vi "LDA_Beam_Alignment.vi"() -> ()   [LabVIEW 2017]
uses:
  Anemometry Sub Vis/Controls/Beam_Type.ctl
  Anemometry Sub Vis/Gen Trav/Traverse_cluster.ctl
  Anemometry Sub Vis/Gen Trav/Spacing.ctl
  Anemometry Sub Vis/Controls/Multi_run_mode.ctl
  Anemometry Sub Vis/Controls/User_Specific_mode.ctl
  Anemometry Sub Vis/Controls/Tunnel_Coordinates.ctl
  Anemometry Sub Vis/Controls/Post_Process.ctl
  Anemometry Sub Vis/Controls/Setup.ctl
  Anemometry Sub Vis/Gen Trav/Trav_mode.ctl
  Anemometry Sub Vis/Globals/Trav_pos_global.vi
  Anemometry Sub Vis/Globals/Meas_global.vi
  Anemometry Sub Vis/Globals/Preference_global.vi
panel:
  in  "Beams to peak":bool[](array[boolean])=[TRUE, TRUE, TRUE, TRUE]
  out "Beam Names":string[](array[string])
  out "Probe is facing...":string
  out "In-Plane Roll (deg)":dbl
  out "Pitch (deg)":dbl
  out "Yaw (deg)":dbl
  out "Vp (Actual Probe dir. vect)":dbl[](array[numeric])
  in  "Mode":T1(ring)
  out "Values Out":dbl[][](array[numeric])
  out "Original Position":dbl[](array[numeric]) format="%.2f"
  in  "Traverse Position":dbl[](array[numeric])=[0.0, 0.0, 0.0] format="%.2f"
  out "Message":string
  in  "Go Back":bool
  in  "OK":bool
  in  "stop":bool
  in  "Working On":T2 items=["Green Unshifted", "Green Shifted", "Blue Unshifted", "Blue Shifted"]
  # "X                 Y              Z"
  # "X                 Y              Z"
  # "Green Unshifted\nGreen Shifted\nBlue Unshifted\nBlue Shifted"
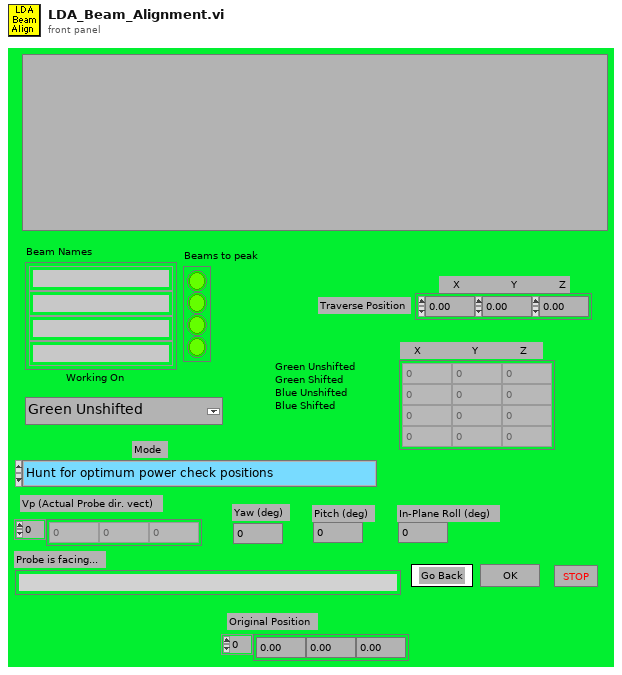
[diagram p1: front panel]
types:
  T1 = enum16{"Hunt for optimum power check positions", "Check Beam powers now", "Peak up beam power using manipulators"}
  T2 = typedef "Beam_Type.ctl" = u16
  T3 = typedef "Traverse_cluster.ctl" = cluster{"Start X":sgl, "Start Y":sgl, "Start Z":sgl, "End X":sgl, "End Y":sgl, "End Z":sgl, "No. of pts.":i32, "Spacing":T4, "Filename":path, "Tunnel Speed":dbl, "Averaging time (min)":dbl, "Extra Commands":string, "Carrier_1 Q (l/min)":dbl, "Carrier_2 Q (l/min)":dbl, "Trace Gas Concentration (%)":dbl, "Specific Arguments":string, "Comments":string, "Row No":i32, "Row Type Selector":T5, "Completion time":string, "Row Duration (mins)":dbl, "No. of Valid pts.":i32, "Meas Setup File":string}
  T4 = typedef "Spacing.ctl" = enum16{"Linear", "Log", "Gauss", "Specified", "N/A"}
  T5 = typedef "Multi_run_mode.ctl" = enum16{"Move Traverse Only", "Set Tunnel Speed Only", "Set Source Only", "Set Measurement Conditions", "Single Measurement", "Vertical Profile", "Lateral Profile", "Longitudinal Profile", "Explore Volume", "Multi-Axis Profile", "Auto Calibrate", "Meas Fast FID Bkgnd", "Check Beam Power", "Scanning Valve Measurement", "Run VI Named:", "Set ADAM Ch", "Wait (minutes)", "Send Message", "Synchronize With:", "Fall Back to this Row", "Turn Off Row Repeating", "Blank Row", "Traverse 3D Volume"}
  T6 = typedef "Tunnel_Coordinates.ctl" = enum16{"Work in Tunnel Coordinates", "Work in Model Coordinates"}
  T7 = typedef "User_Specific_mode.ctl" = enum16{"Check VI only", "Run VI"}
  T8 = typedef "Post_Process.ctl" = enum16{"Take New Data", "Post Process Raw Data File"}
  T9 = enum16{"Load setup from excel file", "Save setup to excel file"}
  T10 = enum16{"Load From Excel File", "Save to Excel File"}
  T11 = typedef "Setup.ctl" = enum16{"Run Program", "Show Setup", "Save Current Setup", "Setup Front Panel"}
  T12 = typedef "Trav_mode.ctl" = enum16{"Move traverse", "Read traverse position", "Teach Position"}
  T13 = typedef "LDA_Beam_Cluster.ctl" = cluster{"Vg1 (Green 1 dir. vect.)":dbl[], "Vg2  (Green 2 dir. vect.)":dbl[], "Vb1 (Blue 1 dir. vect.)":dbl[], "Vb2 (Blue 1 dir. vect.)":dbl[], "Porb (Orb XYZ posn. forced coplanar)":dbl[], "Porb (Orb XYZ posn. - allow skew)":dbl[], "Orb posn. uncertainty, +/- dx, dy, dz":dbl[], "Vp (Actual Probe dir. vect)":dbl[], "Yaw (deg)":dbl, "Pitch (deg)":dbl, "In-Plane Roll (deg)":dbl, "Beam Half Angle (deg)":dbl, "B1 Close P11":dbl[], "B1 Far P12":dbl[], "B2 Close P22":dbl[], "B2 Far P21":dbl[], "Projected Roll (deg)":dbl, "Green Velocity Vector":dbl[], "Blue Velocity Vector":dbl[], "Probe is facing....":string, "Calculation Method":string}
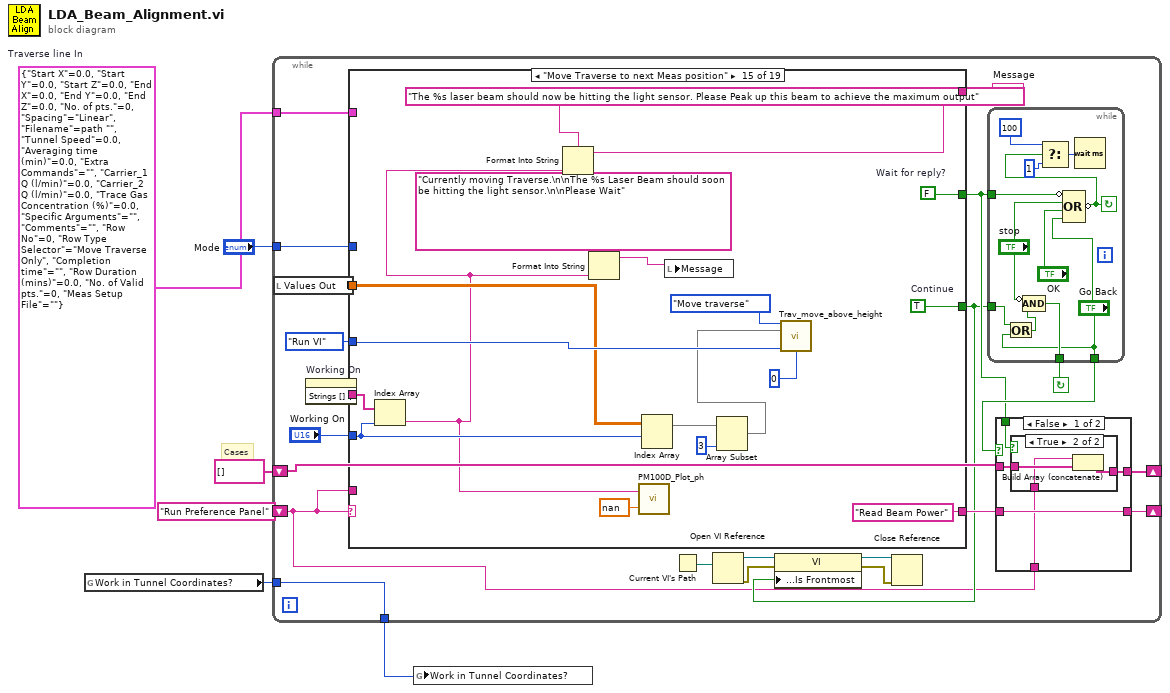
[diagram p0: block diagram]
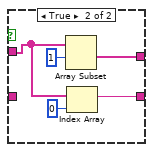
[diagram p3: hidden frame]
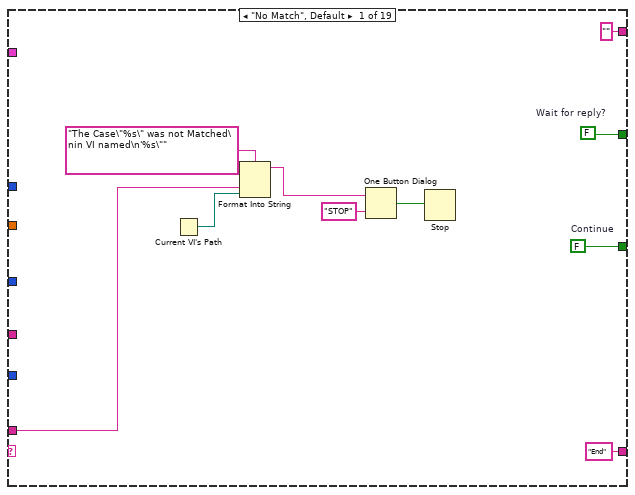
[diagram p4: hidden frame]
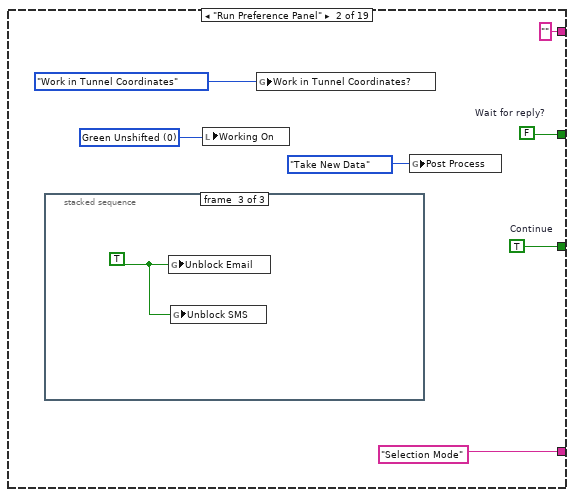
[diagram p5: hidden frame]
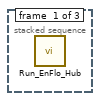
[diagram p6: hidden frame]
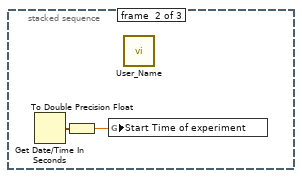
[diagram p7: hidden frame]
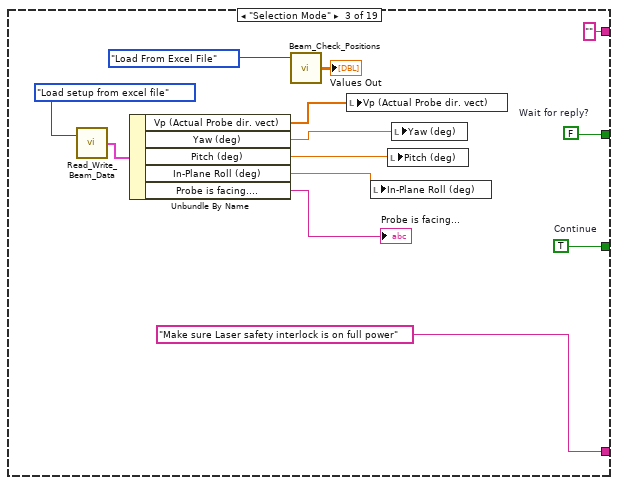
[diagram p8: hidden frame]
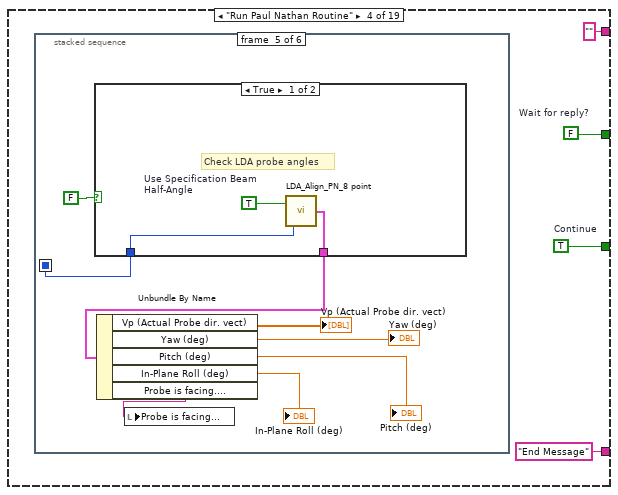
[diagram p9: hidden frame]
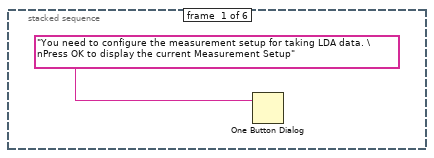
[diagram p10: hidden frame]
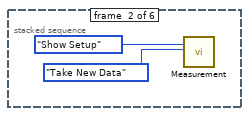
[diagram p11: hidden frame]
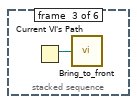
[diagram p12: hidden frame]
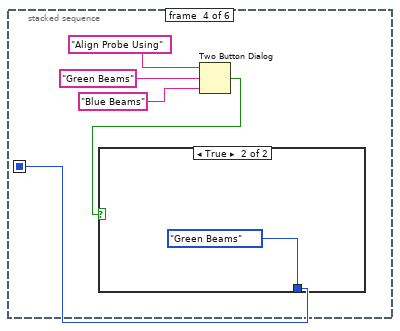
[diagram p13: hidden frame]
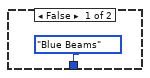
[diagram p14: hidden frame]
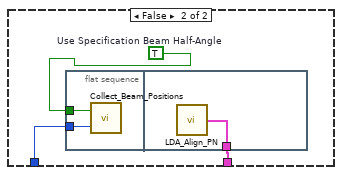
[diagram p15: hidden frame]
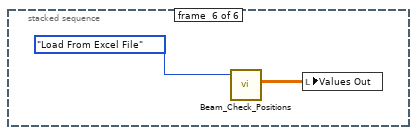
[diagram p16: hidden frame]
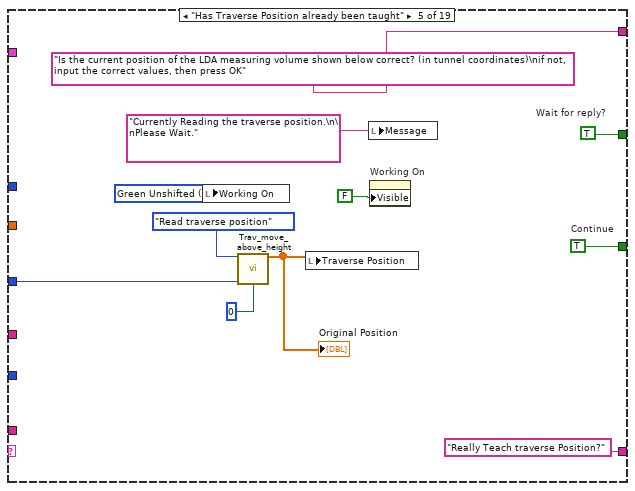
[diagram p17: hidden frame]
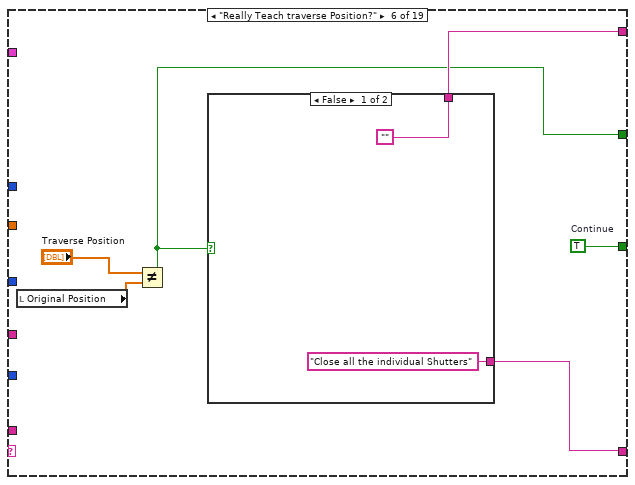
[diagram p18: hidden frame]
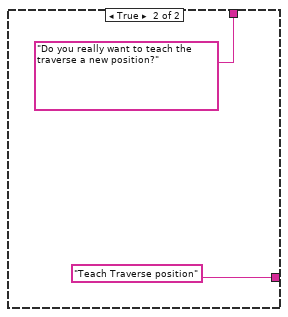
[diagram p19: hidden frame]
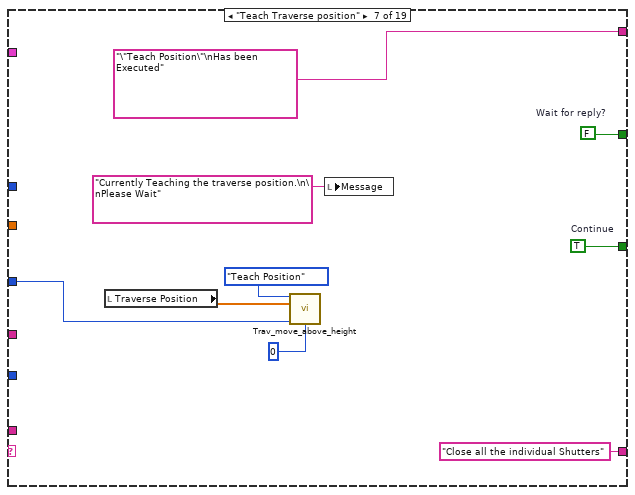
[diagram p20: hidden frame]
diagram:
  w3 = T3 {"Start X"=0.0, "Start Y"=0.0, "Start Z"=0.0, "End X"=0.0, "End Y"=0.0, "End Z"=0.0, "No. of pts."=0, "Spacing"=enum."Linear", "Filename"=path "", "Tunnel Speed"=0.0, "Averaging time (min)"=0.0, "Extra Commands"="", "Carrier_1 Q (l/min)"=0.0, "Carrier_2 Q (l/min)"=0.0, "Trace Gas Concentration (%)"=0.0, "Specific Arguments"="", "Comments"="", "Row No"=0, "Row Type Selector"=enum."Move Traverse Only", "Completion time"="", "Row Duration (mins)"=0.0, "No. of Valid pts."=0, "Meas Setup File"=""}  # Traverse line In
  # "Cases"
  n1 = global read "Trav_pos_global.vi" "Work in Tunnel Coordinates?"() -> (w1:T6)
  n2 = while {
    tunnel: w3 -> [w9]
    tunnel: "Mode" -> [w10]
    shift-left: string[] [] -> [w26]
    shift-right: [w25] -> _
    shift-left: "Run Preference Panel" -> [w8]
    shift-right: [w24] -> _
    tunnel: [w7] -> w2
    tunnel: w1 -> [w7]
    stop <- w28 continue-if-true
    n3 = local read "Values Out"() -> (w11:dbl[][])
    n4 = property on="Working On" class="Ring (strict)"() -> ("Strings []"=w13:string[])  [unwired: 2 in, 2 out]
    n5 = case shown="\"Move Traverse to next Meas position\"" w8 {
      tunnel: [w63 w70 w86 w90 w131 w137 w150 w160 w169 w185 w210 w219 w233 w259 w280 w284 w299 w307 w317] -> w14
      tunnel: ["End" "Selection Mode" "Make sure Laser safety interlock is on full power" "End Message" "Really Teach traverse Position?" w132 "Close all the individual Shutters" "Manually move the traverse using hand wheels" "Read traverse position" w173 w204 "Hunt for optimum power check positions" "End Message" "End Message" "Read Beam Power" "Save measured beam Power" w291 "End Message" "End"] -> w23
      tunnel: [w62 w69 w85 w89 w130 w133 w149 w159 w168 w184 w209 w218 w234 w260 w279 w283 w298 w306 w316] -> w15
      tunnel: ["" "" "" "" "Is the current position of the LDA measuring volume shown below correct? (in tunnel coordinates)\nif not, input the correct values, then press OK" w136 "\"Teach Position\"\nHas been Executed" w153 w162 w170 "Make sure the Laser safety interlock is on full power and all the shutters are open." "Please select which beams you would like to hunt for optimum power check positions for by pressing the green buttons." "" "" w266 w282 w290 "Now open all the individual shutters so all four beam are showing." w310] -> w22
      tunnel: User_Specific_mode."Run VI" ("Simulate/Run") -> [_ _ _ _ w126 _ w145 _ _ w181 _ _ _ _ w276 _ _ _ _]
      tunnel: w13 -> [_ _ _ _ _ _ _ w158 w165 _ w207 w214 w222 _ w271 _ w287 _ _]
      tunnel: "Working On" -> [_ _ _ _ _ _ _ w157 w164 w172 w206 _ _ _ w270 _ w288 _ _]
      tunnel: w11 -> [_ _ _ _ _ _ _ _ _ w171 _ _ _ _ w269 _ w296 _ _]
      tunnel: w10 -> [_ _ _ _ _ _ _ _ _ _ w205 _ _ _ _ _ _ _ w313]
      tunnel: w9 -> [_ _ _ _ _ _ _ _ _ _ _ _ _ w257 _ _ _ _ _]
      tunnel: w8 -> [w54 _ _ _ _ _ _ _ _ _ _ _ _ _ _ _ _ _ _]
      frame "No Match", Default {
        w62 = FALSE  # Wait for reply?
        w63 = FALSE  # Continue
        n6 = Current VI's Path() -> (path=w55:path)
        n7 = Format Into String(format string="The Case\"%s\" was not Matched\nin VI named\n'%s\"" ("Format String"), w54, w55) -> (resulting string=w58:string)  [unwired: 2 in, 1 out]
        n8 = One Button Dialog(message=w58, button name ("OK")="STOP") -> (true=w56:bool)
        n9 = Stop(stop? (T)=w56) -> ()
      }
      frame "Run Preference Panel" {
        w67 = T2 0 items=["Green Unshifted", "Green Shifted", "Blue Unshifted", "Blue Shifted"] ("Beam Type")
        w69 = FALSE  # Wait for reply?
        w70 = TRUE  # Continue
        n10 = stacked-sequence {
          frame #0 {
            n11 = call "Run_EnFlo_Hub.vi"() -> ()  [unwired: 1 in, 7 out]
          }
          frame #1 {
            n12 = Get Date/Time In Seconds() -> (seconds since 1Jan1904=w72:timestamp)
            n13 = To Double Precision Float(number=w72) -> (double precision float=w71:dbl)
            n14 = global write "Meas_global.vi" "Start Time of experiment"(w71) -> ()
            n15 = call "User_Name.vi"() -> ()  [unwired: 1 out]
          }
          frame #2 {
            w73 = TRUE
            n16 = global write "Preference_global.vi" "Unblock Email"(w73) -> ()
            n17 = global write "Preference_global.vi" "Unblock SMS"(w73) -> ()
          }
        }
        n18 = local write "Working On"(w67) -> ()
        n19 = global write "Trav_pos_global.vi" "Work in Tunnel Coordinates?"(Tunnel_Coordinates."Work in Tunnel Coordinates" ("Work in Tunnel Coordinates?")) -> ()
        n20 = global write "Meas_global.vi" "Post Process"(Post_Process."Take New Data" ("Post Process")) -> ()
      }
      frame "Selection Mode" {
        w85 = FALSE  # Wait for reply?
        w86 = TRUE  # Continue
        n21 = call "Read_Write_Beam_Data.vi"("Mode"=T9."Load setup from excel file") -> ("Beam Data Out"=w75:T13)  [unwired: 1 in]
        n22 = Unbundle By Name(w75) -> ("Vp (Actual Probe dir. vect)"=w80:dbl[], "Yaw (deg)"=w77:dbl, "Pitch (deg)"=w78:dbl, "In-Plane Roll (deg)"=w79:dbl, "Probe is facing...."=→"Probe is facing...":string)
        n23 = call "Beam_Check_Positions.vi"("Mode"=T10."Load From Excel File") -> ("Values Out"=→"Values Out":dbl[][])  [unwired: 1 in, 1 out]
        n24 = local write "Vp (Actual Probe dir. vect)"(w80) -> ()
        n25 = local write "In-Plane Roll (deg)"(w79) -> ()
        n26 = local write "Pitch (deg)"(w78) -> ()
        n27 = local write "Yaw (deg)"(w77) -> ()
      }
      frame "Run Paul Nathan Routine" {
        w89 = FALSE  # Wait for reply?
        w90 = TRUE  # Continue
        n28 = stacked-sequence {
          seq-local: [_ _ _ w95 _ _] -> [_ _ _ _ w103 _]
          frame #0 {
            n29 = One Button Dialog(message="You need to configure the measurement setup for taking LDA data. \nPress OK to display the current Measurement Setup") -> ()  [unwired: 1 in, 1 out]
          }
          frame #1 {
            n30 = call "Measurement.vi"("setup"=Setup."Show Setup", "Post Process"=Post_Process."Take New Data") -> ()  [unwired: 16 in, 2 out]
          }
          frame #2 {
            n31 = Current VI's Path() -> (path=w94:path)
            n32 = call "Bring_to_front.vi"("path"=w94) -> ()
          }
          frame #3 {
            n33 = Two Button Dialog(message="Align Probe Using", 1:"Blue Beams" ("F button name (\"Cancel\")"), 2:"Green Beams" ("T button name (\"OK\")")) -> (T button?=w96:bool)
            n34 = case shown="True" w96 {
              tunnel: [enum16{"Green Beams", "Blue Beams"}."Blue Beams" ("Align Probe Using") enum16{"Green Beams", "Blue Beams"}."Green Beams" ("Align Probe Using")] -> w95
              frame False {
              }
              frame True {
              }
            }
          }
          frame #4 {
            n35 = case shown="True" FALSE ("Case Constant\n(See Context Help)") {
              tunnel: [w111 w113] -> w109
              tunnel: w103 -> [w110 w115]
              frame True {
                w112 = TRUE  # Use Specification Beam Half-Angle
                # "Check LDA probe angles"
                n36 = call "LDA_Align_PN_8 point.vi"("Align Probe Using"=w110, "Use Specification Beam Half-Angle"=w112) -> ("Beam Data"=w111:T13)
              }
              frame False {
                w114 = TRUE  # Use Specification Beam Half-Angle
                n37 = flat-sequence {
                  tunnel: w115 -> [w117]
                  tunnel: w114 -> [w116]
                  tunnel: [w118] -> w113
                  frame #0 {
                    n38 = call "Collect_Beam_Positions.vi"("Align Probe Using"=w117, "Use Specification Beam Half-Angle"=w116) -> ()  [unwired: 1 out]
                  }
                  frame #1 {
                    n39 = call "LDA_Align_PN.vi"() -> ("Beam Data"=w118:T13)  [unwired: 2 in]
                  }
                }
              }
            }
            n40 = Unbundle By Name(w109) -> ("Vp (Actual Probe dir. vect)"=→"Vp (Actual Probe dir. vect)":dbl[], "Yaw (deg)"=→"Yaw (deg)":dbl, "Pitch (deg)"=→"Pitch (deg)":dbl, "In-Plane Roll (deg)"=→"In-Plane Roll (deg)":dbl, "Probe is facing...."=w104:string)
            n41 = local write "Probe is facing..."(w104) -> ()
          }
          frame #5 {
            n42 = call "Beam_Check_Positions.vi"("Mode"=T10."Load From Excel File") -> ("Values Out"=w119:dbl[][])  [unwired: 1 in, 1 out]
            n43 = local write "Values Out"(w119) -> ()
          }
        }
      }
      frame "Has Traverse Position already been taught" {
        w124 = T2 0 items=["Green Unshifted", "Green Shifted", "Blue Unshifted", "Blue Shifted"] ("Beam Type")
        w130 = TRUE  # Wait for reply?
        w131 = TRUE  # Continue
        n44 = local write "Working On"(w124) -> ()
        n45 = call "Trav_move_above_height.vi"("Mode"=Trav_mode."Read traverse position", "Simulate/Run"=w126, "Currently on Point"=0) -> ("Trav Position achieved"=w125:sgl[])  [unwired: 10 in, 2 out]
        "Original Position" <- w125
        n46 = local write "Traverse Position"(w125) -> ()
        n47 = local write "Message"("Currently Reading the traverse position.\n\nPlease Wait." ("Message")) -> ()
        n48 = property on="Working On" class="Ring (strict)"("Visible"=FALSE ("Write Attribute")) -> ()  [unwired: 2 in, 2 out]
      }
      frame "Really Teach traverse Position?" {
        w137 = TRUE  # Continue
        n49 = local read "Original Position"() -> (w135:dbl[])
        n50 = Not Equal?(x="Traverse Position", y=w135) -> (x != y?=w133:bool)
        n51 = case shown="False" w133 {
          tunnel: ["" "Do you really want to teach the traverse a new position?"] -> w136
          tunnel: ["Close all the individual Shutters" "Teach Traverse position"] -> w132
          frame False {
          }
          frame True {
          }
        }
      }
      frame "Teach Traverse position" {
        w149 = FALSE  # Wait for reply?
        w150 = TRUE  # Continue
        n52 = local read "Traverse Position"() -> (w144:dbl[])
        n53 = call "Trav_move_above_height.vi"("Mode"=Trav_mode."Teach Position", "New Position"=w144, "Simulate/Run"=w145, "Currently on Point"=0) -> ()  [unwired: 9 in, 3 out]
        n54 = local write "Message"("Currently Teaching the traverse position.\n\nPlease Wait" ("Message")) -> ()
      }
      frame "Close all the individual Shutters" {
        w159 = TRUE  # Wait for reply?
        w160 = TRUE  # Continue
        n55 = Index Array(array=w158, index=w157) -> (element=w156:string)
        n56 = Format Into String(format string="Close all the individual shutters except for the %s laser beam.", w156) -> (resulting string=w153:string)  [unwired: 2 in, 1 out]
        n57 = property on="Working On" class="Ring (strict)"("Visible"=TRUE ("Write Attribute"), "Disabled"=u8 0 ("Write Attribute")) -> ()  [unwired: 2 in, 2 out]
      }
      frame "Manually move the traverse using hand wheels" {
        w168 = TRUE  # Wait for reply?
        w169 = TRUE  # Continue
        n58 = Index Array(array=w165, index=w164) -> (element=w166:string)
        n59 = property on="Working On" class="Ring (strict)"("Disabled"=u8 1 ("Write Attribute")) -> ()  [unwired: 2 in, 2 out]
        n60 = Format Into String(format string="Go into the tunnel and manually move the traverse using the hand wheels so that the %s laser beam is pointing at the center of the light sensor.\n", w166) -> (resulting string=w162:string)  [unwired: 2 in, 1 out]
      }
      frame "Read traverse position" {
        w175 = T2 3 items=["Green Unshifted", "Green Shifted", "Blue Unshifted", "Blue Shifted"] ("Beam Type")
        w170 = "Currently Reading the traverse Position.\n\nPlease Wait"
        w184 = FALSE  # Wait for reply?
        w185 = TRUE  # Continue
        n61 = To Long Integer(number=w172) -> (32bit integer=w180:i32)
        n62 = call "Trav_move_above_height.vi"("Mode"=Trav_mode."Read traverse position", "Simulate/Run"=w181, "Currently on Point"=0) -> ("Trav Position achieved"=w179:sgl[])  [unwired: 10 in, 2 out]
        n63 = for {
          N: 4 -> [_]
          tunnel: w171 -> [w196]
          tunnel: w180 -> [w194]
          tunnel: [w192] -> w176 mode=indexing
          tunnel: w179 -> [w190]
          i -> [w195]
          n64 = Index Array(array=w196, index (row)=w195) -> (element=w191:dbl[])  [unwired: 1 in]
          n65 = Equal?(x=w195, y=w194) -> (x = y?=w193:bool)
          n66 = case shown="True" w193 {
            tunnel: [w197 w200] -> w192
            tunnel: w191 -> [w197 w202]
            tunnel: w190 -> [_ w198]
            frame False {
            }
            frame True {
              n67 = Index Array(array=w202, index=3 ("Index")) -> (element=w199:dbl)
              n68 = Build Array (concatenate)(w198, w199) -> (w200:dbl[])
            }
          }
        }
        n69 = Equal?(x=w172, y=w175) -> (x = y?=w174:bool)
        n70 = case shown="False" w174 {
          tunnel: ["Close all the individual Shutters" "Open all individual laser shutters again"] -> w173
          tunnel: w172 -> [w187 _]
          frame False {
            n71 = Increment(x=w187) -> (x+1=w188:T2)
            n72 = local write "Working On"(w188) -> ()
          }
          frame True {
          }
        }
        n73 = local write "Values Out"(w176) -> ()
        n74 = local write "Message"(w170) -> ()
        n75 = call "Beam_Check_Positions.vi"("Values"=w176, "Mode"=T10."Save to Excel File") -> ()  [unwired: 2 out]
      }
      frame "Make sure Laser safety interlock is on full power" {
        w209 = TRUE  # Wait for reply?
        w210 = TRUE  # Continue
        n76 = Index Array(array=w207, index=w206) -> ()  [unwired: 1 out]
        n77 = property on="Working On" class="Ring (strict)"("Disabled"=u8 1 ("Write Attribute")) -> ()  [unwired: 2 in, 2 out]
        n78 = case shown="\"Hunt for optimum power check positions\"" w205 {
          tunnel: ["Find Peak for which beams?" "Check Beam powers now" "Move Traverse to next Meas position"] -> w204
          frame "Hunt for optimum power check positions" {
          }
          frame "Check Beam powers now" {
          }
          frame "Peak up beam power using manipulators" {
          }
        }
      }
      frame "Find Peak for which beams?" {
        w218 = TRUE  # Wait for reply?
        w219 = TRUE  # Continue
        n79 = property on="Working On" class="Ring (strict)"("Disabled"=u8 1 ("Write Attribute")) -> ()  [unwired: 2 in, 2 out]
        "Beam Names" <- w214
      }
      frame "Hunt for optimum power check positions" {
        w234 = FALSE  # Wait for reply?
        w233 = TRUE  # Continue
        w239 = T3 {"Start X"=0.0, "Start Y"=0.0, "Start Z"=0.0, "End X"=0.0, "End Y"=0.0, "End Z"=0.0, "No. of pts."=0, "Spacing"=enum."Linear", "Filename"=path "", "Tunnel Speed"=0.0, "Averaging time (min)"=0.0, "Extra Commands"="", "Carrier_1 Q (l/min)"=0.0, "Carrier_2 Q (l/min)"=0.0, "Trace Gas Concentration (%)"=0.0, "Specific Arguments"="", "Comments"="", "Row No"=0, "Row Type Selector"=enum."Move Traverse Only", "Completion time"="", "Row Duration (mins)"=0.0, "No. of Valid pts."=0, "Meas Setup File"=""}  # Traverse line In
        w225 = 0.85 ("y")
        n80 = local read "Vp (Actual Probe dir. vect)"() -> (w231:dbl[])
        n81 = for {
          shift-right: [w243] -> w221
          shift-left: "; " -> [w242]
          tunnel: "Beams to peak" -> [w244] mode=indexing
          tunnel: w222 -> [w241] mode=indexing
          n82 = case shown="True" w244 {
            tunnel: [w245 w249] -> w243
            tunnel: w242 -> [w245 w248]
            tunnel: w241 -> [_ w247]
            frame False {
            }
            frame True {
              n83 = Concatenate Strings(w248, w247, ";  " ("string")) -> (w249:string)
            }
          }
        }
        n84 = Absolute Value(x=w231) -> (abs(x)=w230:dbl[])
        n85 = Array To Cluster(array=w230) -> (cluster=w229:cluster{"[0]":dbl, "[1]":dbl, "[2]":dbl})
        n86 = Unbundle(w229) -> ("[0]"=w228:dbl, "[1]"=w226:dbl)  [unwired: 1 out]
        n87 = Greater?(x=w228, y=w225) -> (0:w227:bool)
        n88 = case shown="True" w227 {
          tunnel: [w253 "X Axis Fixed"] -> w240
          tunnel: w226 -> [w252 _]
          tunnel: w225 -> [w251 _]
          frame False {
            n89 = Greater?(x=w252, y=w251) -> (0:w250:bool)
            n90 = case shown="False" w250 {
              tunnel: ["Z Axis Fixed" "Y Axis Fixed"] -> w253
              frame False {
              }
              frame True {
              }
            }
          }
          frame True {
          }
        }
        n91 = Concatenate Strings("First Argument;" ("string"), w240, w221) -> (w238:string)
        n92 = Bundle By Name(cluster=w239, "Specific Arguments"=w238) -> (w237:T3)
        n93 = call "Find_Beam_Max_Pos.vi"("Mode"=User_Specific_mode."Run VI", "Traverse line In"=w237) -> ()  [unwired: 4 out]
      }
      frame "Check Beam powers now" {
        w260 = FALSE  # Wait for reply?
        w259 = TRUE  # Continue
        n94 = call "Check_Beam_Powers.vi"("Mode"=User_Specific_mode."Run VI", "Traverse line In"=w257) -> ()  [unwired: 1 in, 3 out]
      }
      frame "Move Traverse to next Meas position" {
        w279 = FALSE  # Wait for reply?
        w280 = TRUE  # Continue
        n95 = Index Array(array=w271, index=w270) -> (element=w264:string)
        n96 = Format Into String(format string="The %s laser beam should now be hitting the light sensor. Please Peak up this beam to achieve the maximum output", w264) -> (resulting string=w266:string)  [unwired: 2 in, 1 out]
        n97 = Format Into String(format string="Currently moving Traverse.\n\nThe %s Laser Beam should soon be hitting the light sensor.\n\nPlease Wait", w264) -> (resulting string=w268:string)  [unwired: 2 in, 1 out]
        n98 = call "PM100D_Plot_ph.vi"("Meas Time (s)"=nan, "Beam Name"=w264) -> ()  [unwired: 2 out]
        n99 = Index Array(array=w269, index (row)=w270) -> (element=w275:dbl[])  [unwired: 1 in]
        n100 = local write "Message"(w268) -> ()
        n101 = Array Subset(array=w275, length=3 ("Array Length")) -> (w273:dbl[])  [unwired: 1 in]
        n102 = call "Trav_move_above_height.vi"("Mode"=Trav_mode."Move traverse", "New Position"=w273, "Simulate/Run"=w276, "Currently on Point"=0) -> ()  [unwired: 9 in, 3 out]
      }
      frame "Read Beam Power" {
        w282 = "Currently Reading the Beam Power\n\nPlease Wait"
        w283 = FALSE  # Wait for reply?
        w284 = TRUE  # Continue
        n103 = local write "Message"(w282) -> ()
      }
      frame "Save measured beam Power" {
        w293 = T2 3 items=["Green Unshifted", "Green Shifted", "Blue Unshifted", "Blue Shifted"] ("Beam Type")
        w290 = "Writing Beam Power to file"
        w298 = FALSE  # Wait for reply?
        w299 = TRUE  # Continue
        n104 = Index Array(array=w287, index=w288) -> (element=w286:string)
        n105 = Equal?(x=w288, y=w293) -> (x = y?=w292:bool)
        n106 = call "PM100D_Single_Value_ph.vi"("Averaging Period (s)"=3.0, "Beam Name"=w286) -> ("Light Power mW"=w289:dbl)  [unwired: 1 out]
        n107 = case shown="False" w292 {
          tunnel: ["Move Traverse to next Meas position" "End Message"] -> w291
          tunnel: w288 -> [w302 _]
          frame False {
            n108 = Increment(x=w302) -> (x+1=w301:T2)
            n109 = local write "Working On"(w301) -> ()
          }
          frame True {
          }
        }
        n110 = Replace Array Subset(array=w296, new element=w289, index (row)=w288, index (col)=3 ("Index")) -> (w294:dbl[][])
        n111 = local write "Message"(w290) -> ()
        n112 = local write "Values Out"(w294) -> ()
        n113 = call "Beam_Check_Positions.vi"("Values"=w294, "Mode"=T10."Save to Excel File") -> ()  [unwired: 2 out]
      }
      frame "Open all individual laser shutters again" {
        w306 = TRUE  # Wait for reply?
        w307 = TRUE  # Continue
      }
      frame "End Message" {
        w316 = FALSE  # Wait for reply?
        w317 = FALSE  # Continue
        n114 = property on="Mode" class="Enum (strict)"() -> ("Strings []"=w314:string[])  [unwired: 2 in, 2 out]
        n115 = Index Array(array=w314, index=w313) -> (element=w312:string)
        n116 = Format Into String(format string="%s\nhas now been completed" ("Format String"), w312) -> (resulting string=w310:string)  [unwired: 2 in, 1 out]
        n117 = call "Beam_Check_Positions.vi"("Mode"=T10."Load From Excel File") -> ("Values Out"=w308:dbl[][])  [unwired: 1 in, 1 out]
        n118 = local write "Values Out"(w308) -> ()
      }
    }
    "Message" <- w22
    n119 = Current VI's Path() -> (path=w20:path)
    n120 = Open VI Reference(vi path=w20) -> (vi reference=w19:refnum<vi>, error out=w18:errorcluster)  [unwired: 1 in, 4 out]
    n121 = property class="VI"(reference=w19, error in=w18, "Front Panel Window:Is Frontmost"=w14) -> (reference out=w17:refnum<vi>, error out=w16:errorcluster)
    n122 = Close Reference(reference=w17, error in (no error)=w16) -> ()  [unwired: 1 out]
    n123 = while {
      tunnel: ["Go Back"] -> w27
      tunnel: [w36] -> w28
      tunnel: w14 -> [w35]
      tunnel: w15 -> [w38]
      stop <- w32 continue-if-true
      n124 = Or(x=w35, y="Go Back") -> (x .or. y?=w33:bool)
      n125 = Compound Arithmetic op=AND(invert "stop", w33) -> (w36:bool)
      n126 = Compound Arithmetic op=OR(invert w38, "stop", "OK", "Go Back") -> (invert w32:bool)
      n127 = Select(t=u32 100 ("millisecond timer value"), s=w32, f=u32 1) -> (s? t:f=w29:u32)
      n128 = Wait (ms)(milliseconds to wait=w29) -> ()  [unwired: 1 out]
    }
    n129 = case shown="False" w27 {
      tunnel: w26 -> [w44 w49]
      tunnel: [w43 w50] -> w25
      tunnel: w8 -> [w41 _]
      tunnel: [w42 w51] -> w24
      tunnel: w23 -> [w42 _]
      tunnel: w15 -> [w40 _]
      frame False {
        n130 = case shown="True" w40 {
          tunnel: w44 -> [w45 w48]
          tunnel: [w45 w47] -> w43
          tunnel: w41 -> [_ w46]
          frame False {
          }
          frame True {
            n131 = Build Array (concatenate)(w46, w48) -> (w47:string[])
          }
        }
      }
      frame True {
        n132 = Array Subset(array=w49, index=1 ("Array Index")) -> (w50:string[])  [unwired: 1 in]
        n133 = Index Array(array=w49, index=0 ("Index")) -> (element=w51:string)
      }
    }
  }
  n134 = global write "Trav_pos_global.vi" "Work in Tunnel Coordinates?"(w2) -> ()
